vi "Fetch.vi"(8 "error in (no error)":errorcluster, 10 "Message in":refnum<class "FetchMessage.lvclass">, 11 "Template in":refnum<class "Template.lvclass">) -> (0 "error out":errorcluster, 3 "Template out":refnum<class "Template.lvclass">)   [LabVIEW 2012, in "Template.lvclass"]
doc: "The fetch method processes the command 'fetch'.\n\nThe command 'fetch' is used for receiving various forms of data."
uses:
  Template.lvclass
  <vilib>/Distrio/Murmex/FetchMessage/FetchMessage.lvclass
  <vilib>/Distrio/Murmex/Murmex/Murmex.lvclass
  <vilib>/Waveform/DWDTOps.llb/DWDT Binary U32 to Digital.vi
panel:
  out "anlg waveforms":waveform(i32)[](array[waveform])
  out "dig waveforms":digitalwaveform[](array[waveform])
  # "This method is called when the FETCH\ntrigger is sent. \n\nOverride this method when your component needs to\nrespond to this trigger. \n\nCall parent for proper implementation"
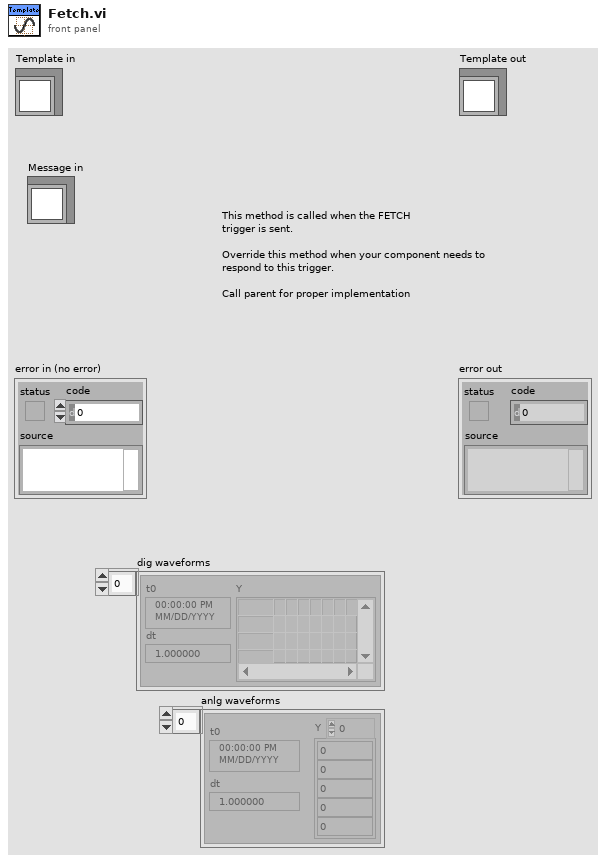
[diagram p1: front panel]
types:
  T1 = typedef "Murmex.lvlib/FetchMessage.lvclass/Channel data cluster.ctl" = cluster{"channel id":i32, "data UInt8":u8[], "data type":T2, "dimensions":i32[], "physical units":T3[], "waveform dt":dbl, "waveform":T4}
  T2 = typedef "Murmex.lvlib/Murmex.lvclass/data_type_enum.ctl" = enum16{"Float128", "Float64", "Float32", "Int64", "Int32", "Int16", "Int8", "UInt64", "UInt32", "UInt16", "UInt8", "Boolean", "String"}
  T3 = typedef "Murmex.lvlib/Murmex.lvclass/Physical Units.ctl" = cluster{"Base Units":enum16{"radian", "steradian", "second", "meter", "kilogram", "ampere", "kelvin", "mole", "candela"}, "Exponent":i16}
  T4 = typedef "Murmex.lvlib/Murmex.lvclass/waveform_type_enum.ctl" = enum16{"no waveform", "analog", "digital"}
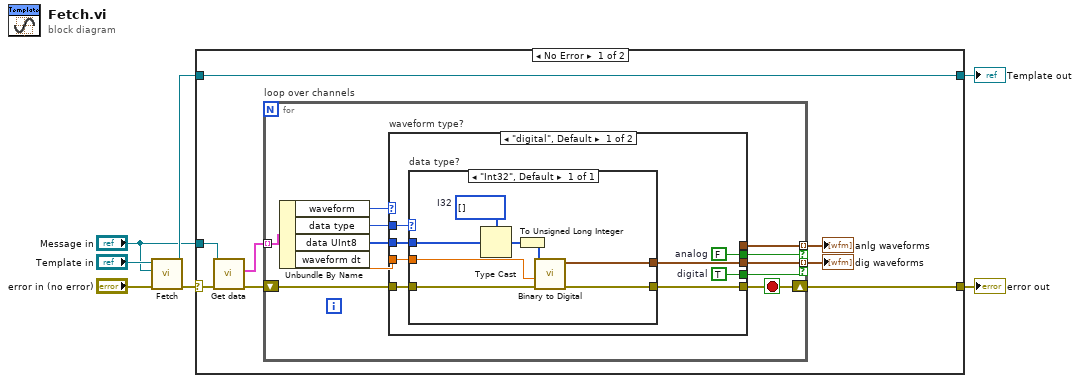
[diagram p0: block diagram]
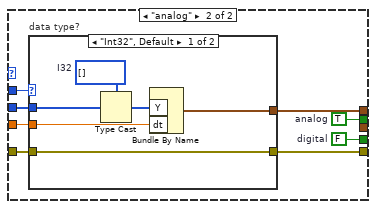
[diagram p2: hidden frame]
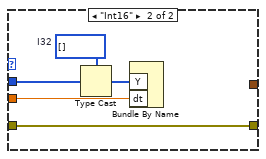
[diagram p3: hidden frame]
diagram:
  n1 = call-parent "Fetch.vi"("error in (no error)"="error in (no error)", "Message in"="Message in", "Murmex in"="Template in") -> ("error out"=w5:errorcluster, "Murmex out"=w2:refnum<class "Template.lvclass">)  [unwired: 7 in]
  n2 = case shown="No Error" w5 {
    selector: w5 -> [w14 w63]
    tunnel: [w10 w63] -> w4
    tunnel: [w13 w62] -> w3
    tunnel: w2 -> [w13 w62]
    tunnel: "Message in" -> [w15 _]
    frame No Error {
      n3 = call <vilib>:"Get data.vi"("error in (no error)"=w14, "FetchMessage.lvclass"=w15) -> ("error out"=w11:errorcluster, "data (channels)"=w12:T1[])  [unwired: 7 in, 1 out]
      n4 = for "loop over channels" {
        tunnel: w12 -> [w26] mode=indexing
        tunnel: [w22] -> w9 mode=indexing if=w18
        shift-right: [w20] -> w10
        shift-left: w11 -> [w21]
        tunnel: [w17] -> w8 mode=indexing if=w16
        stop <- w20 stop-if-true
        n5 = Unbundle By Name(w26) -> ("waveform"=w19:T4, "data type"=w25:T2, "data UInt8"=w24:u8[], "waveform dt"=w23:dbl)
        n6 = case "waveform type?" shown="\"digital\", Default" w19 {
          tunnel: w25 -> [w34 w50]
          tunnel: w24 -> [w33 w49]
          tunnel: w23 -> [w32 w48]
          tunnel: [w31 _] -> w22
          tunnel: w21 -> [w30 w47]
          tunnel: [w29 w46] -> w20
          tunnel: [w28 w43] -> w18
          tunnel: [_ w45] -> w17
          tunnel: [w27 w44] -> w16
          frame "digital", Default {
            w27 = FALSE  # analog
            w28 = TRUE  # digital
            n7 = case "data type?" shown="\"Int32\", Default" w34 {
              tunnel: w33 -> [w42]
              tunnel: w32 -> [w39]
              tunnel: [w37] -> w31
              tunnel: w30 -> [w36]
              tunnel: [w35] -> w29
              frame "Int32", Default {
                w41 = i32[] []  # I32
                n8 = Type Cast(type=w41, x=w42) -> (*(type *) &x=w40:i32[])
                n9 = To Unsigned Long Integer(number=w40) -> (unsigned 32bit integer=w38:u32[])
                n10 = call-poly <vilib>:"Binary to Digital.vi"("error in (no error)"=w36, "sample rate"=w39, "binary array"=w38) -> ("error out"=w35:errorcluster, "digital waveform"=w37:digitalwaveform)  [unwired: 7 in]
              }
            }
          }
          frame "analog" {
            w43 = FALSE  # digital
            w44 = TRUE  # analog
            n11 = case "data type?" shown="\"Int32\", Default" w50 {
              tunnel: w49 -> [w56 w61]
              tunnel: w48 -> [w52 w57]
              tunnel: w47 -> [w54 w59]
              tunnel: [w54 w59] -> w46
              tunnel: [w51 _] -> w45
              frame "Int32", Default {
                w55 = i32[] []  # I32
                n12 = Type Cast(type=w55, x=w56) -> (*(type *) &x=w53:i32[])
                n13 = Bundle By Name("Y"=w53, "dt"=w52) -> (w51:waveform(i32))  [unwired: 1 in]
              }
              frame "Int16" {
                w60 = i32[] []  # I32
                n14 = Type Cast(type=w60, x=w61) -> (*(type *) &x=w58:i32[])
                n15 = Bundle By Name("Y"=w58, "dt"=w57) -> ()  [unwired: 1 in, 1 out]
              }
            }
          }
        }
      }
      "dig waveforms" <- w9
      "anlg waveforms" <- w8
    }
    frame Error {
    }
  }
  "error out" <- w4
  "Template out" <- w3
